vi "_PC_Toolbar enable_toolbar_buttons.vi"(0 "Disabled":T1(ring), 1 "Function":enum16{"Save reference", "Operation"}(ring)=enum."Operation", 2 "Cluster control array":refnum<vi>[](array[refnum]), 3 "error in (no error)":errorcluster) -> (9 "error out":errorcluster)   [LabVIEW 2018]
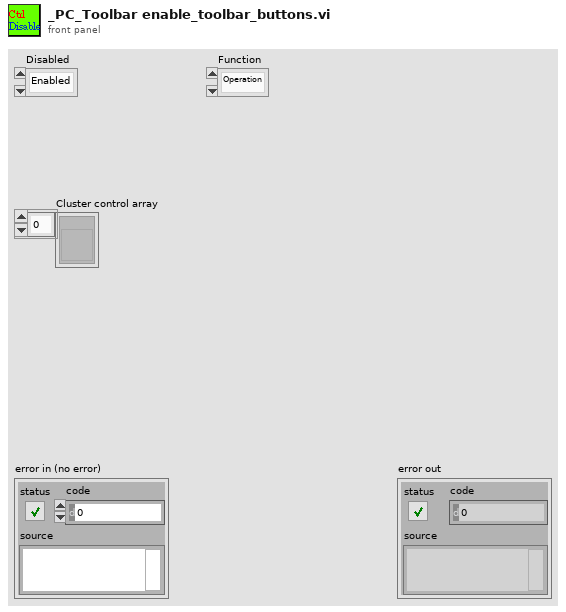
[diagram p1: front panel]
types:
  T1 = enum8{"Enabled", "Disabled", "Disabled and Grayed Out"}
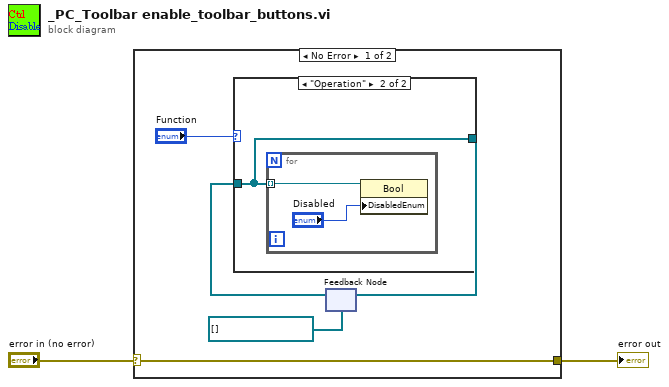
[diagram p0: block diagram]
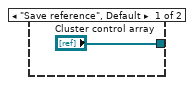
[diagram p2: hidden frame]
diagram:
  n1 = case shown="No Error" "error in (no error)" {
    selector: "error in (no error)" -> [w3 w12]
    tunnel: [w3 w12] -> w1
    frame No Error {
      n2 = feedback #1(refnum<vi>[] [] ("Cluster control array")) -> (w5:refnum<vi>[])
      n3 = case shown="\"Operation\"" "Function" {
        tunnel: ["Cluster control array" w9] -> w6
        tunnel: w5 -> [_ w9]
        frame "Save reference", Default {
        }
        frame "Operation" {
          n4 = for {
            tunnel: w9 -> [w11] mode=indexing
            n5 = property class="Bool"(reference=w11, "DisabledEnum"="Disabled") -> ()  [unwired: 1 in, 2 out]
          }
        }
      }
      n6 = feedback-in #1(w6) -> ()
    }
    frame Error {
    }
  }
  "error out" <- w1
